vi "Backward Number Split.vi"(0 "number as string":string) -> (1 "string start":string, 2 "string rest":string)   [LabVIEW 2018, in "NI_Gmath.lvlib"]
uses:
  NI_Gmath.lvlib
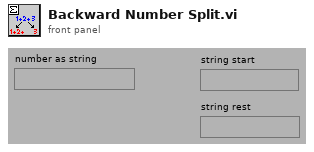
[diagram p1: front panel]
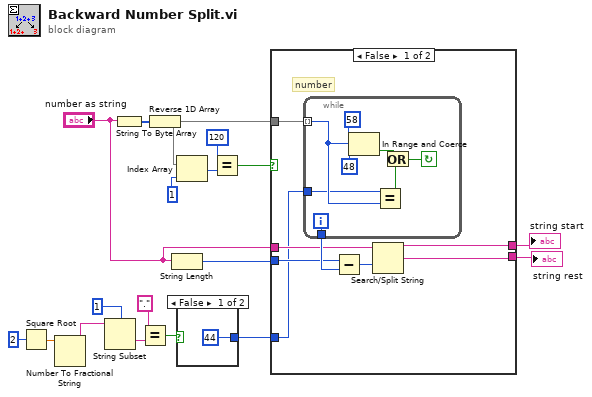
[diagram p0: block diagram]
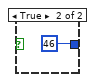
[diagram p2: hidden frame]
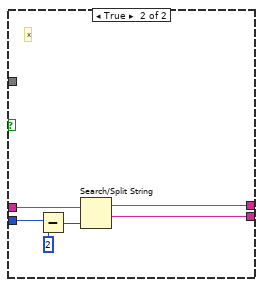
[diagram p3: hidden frame]
diagram:
  w7 = 1
  n1 = Square Root(x=2) -> (sqrt(x)=w5:dbl)
  n2 = Number To Fractional String(number=w5) -> (F-format string=w8:string)  [unwired: 3 in]
  n3 = String Subset(string=w8, offset (0)=w7, length (rest)=w7) -> (substring=w4:string)
  n4 = String To Byte Array(string="number as string") -> (unsigned byte array=w18:u8[])
  n5 = Equal?(x=".", y=w4) -> (x = y?=w2:bool)
  n6 = Reverse 1D Array(array=w18) -> (reversed array=w17:u8[])
  n7 = String Length(string="number as string") -> (length=w12:i32)
  n8 = Index Array(array=w17, index=1) -> (element=w14:u8)
  n9 = case shown="False" w2 {
    tunnel: [44 46] -> w1
    frame False {
    }
    frame True {
    }
  }
  n10 = Equal?(x=120, y=w14) -> (x = y?=w13:bool)
  n11 = case shown="False" w13 {
    tunnel: w12 -> [w26 w42]
    tunnel: "number as string" -> [w25 w37]
    tunnel: [w23 w39] -> w10
    tunnel: [w22 w38] -> w9
    tunnel: w17 -> [w28 _]
    tunnel: w1 -> [w21 _]
    frame False {
      # "number"
      n12 = while {
        tunnel: w21 -> [w29]
        tunnel: [w30] -> w27
        tunnel: w28 -> [w34] mode=indexing
        i -> [w30]
        stop <- w31 continue-if-true
        n13 = In Range and Coerce(upper limit=58, x=w34, lower limit=48) -> (In Range?=w33:bool)  [unwired: 1 out]
        n14 = Equal?(x=w29, y=w34) -> (x = y?=w32:bool)
        n15 = Or(x=w33, y=w32) -> (x .or. y?=w31:bool)
      }
      n16 = Subtract(x=w26, y=w27) -> (x-y=w24:i32)
      n17 = Search/Split String(string=w25, offset (0)=w24) -> (substring before match=w23:string, match + rest of string=w22:string)  [unwired: 1 in, 1 out]
    }
    frame True {
      # "x"
      n18 = Subtract(x=w42, y=2) -> (x-y=w40:i32)
      n19 = Search/Split String(string=w37, offset (0)=w40) -> (substring before match=w39:string, match + rest of string=w38:string)  [unwired: 1 in, 1 out]
    }
  }
  "string start" <- w10
  "string rest" <- w9
